vi "Digital Output.vi"(8 "error in":errorcluster, 11 "DAQmx OutPut Setting":T1) -> (0 "error out":errorcluster, 1 "Exit":bool)   [LabVIEW 2015]
uses:
  <vilib>/DAQmx/write.llb/DAQmx Write (Digital 2D Bool NChan 1Samp NLine).vi
  <vilib>/DAQmx/write.llb/DAQmx Write (Digital 1D Bool 1Chan 1Samp).vi
  <vilib>/DAQmx/create/channels.llb/DAQmx Create Channel (DO-Digital Output).vi
  Galobal variable_TI.vi
  <vilib>/DAQmx/miscellaneous.llb/DAQmx Fill In Error Info.vi
panel:
  out "array":tag[](array[tag])
  out "*(type *) &x":tag
  out "Digital Output":bool[](array[boolean])
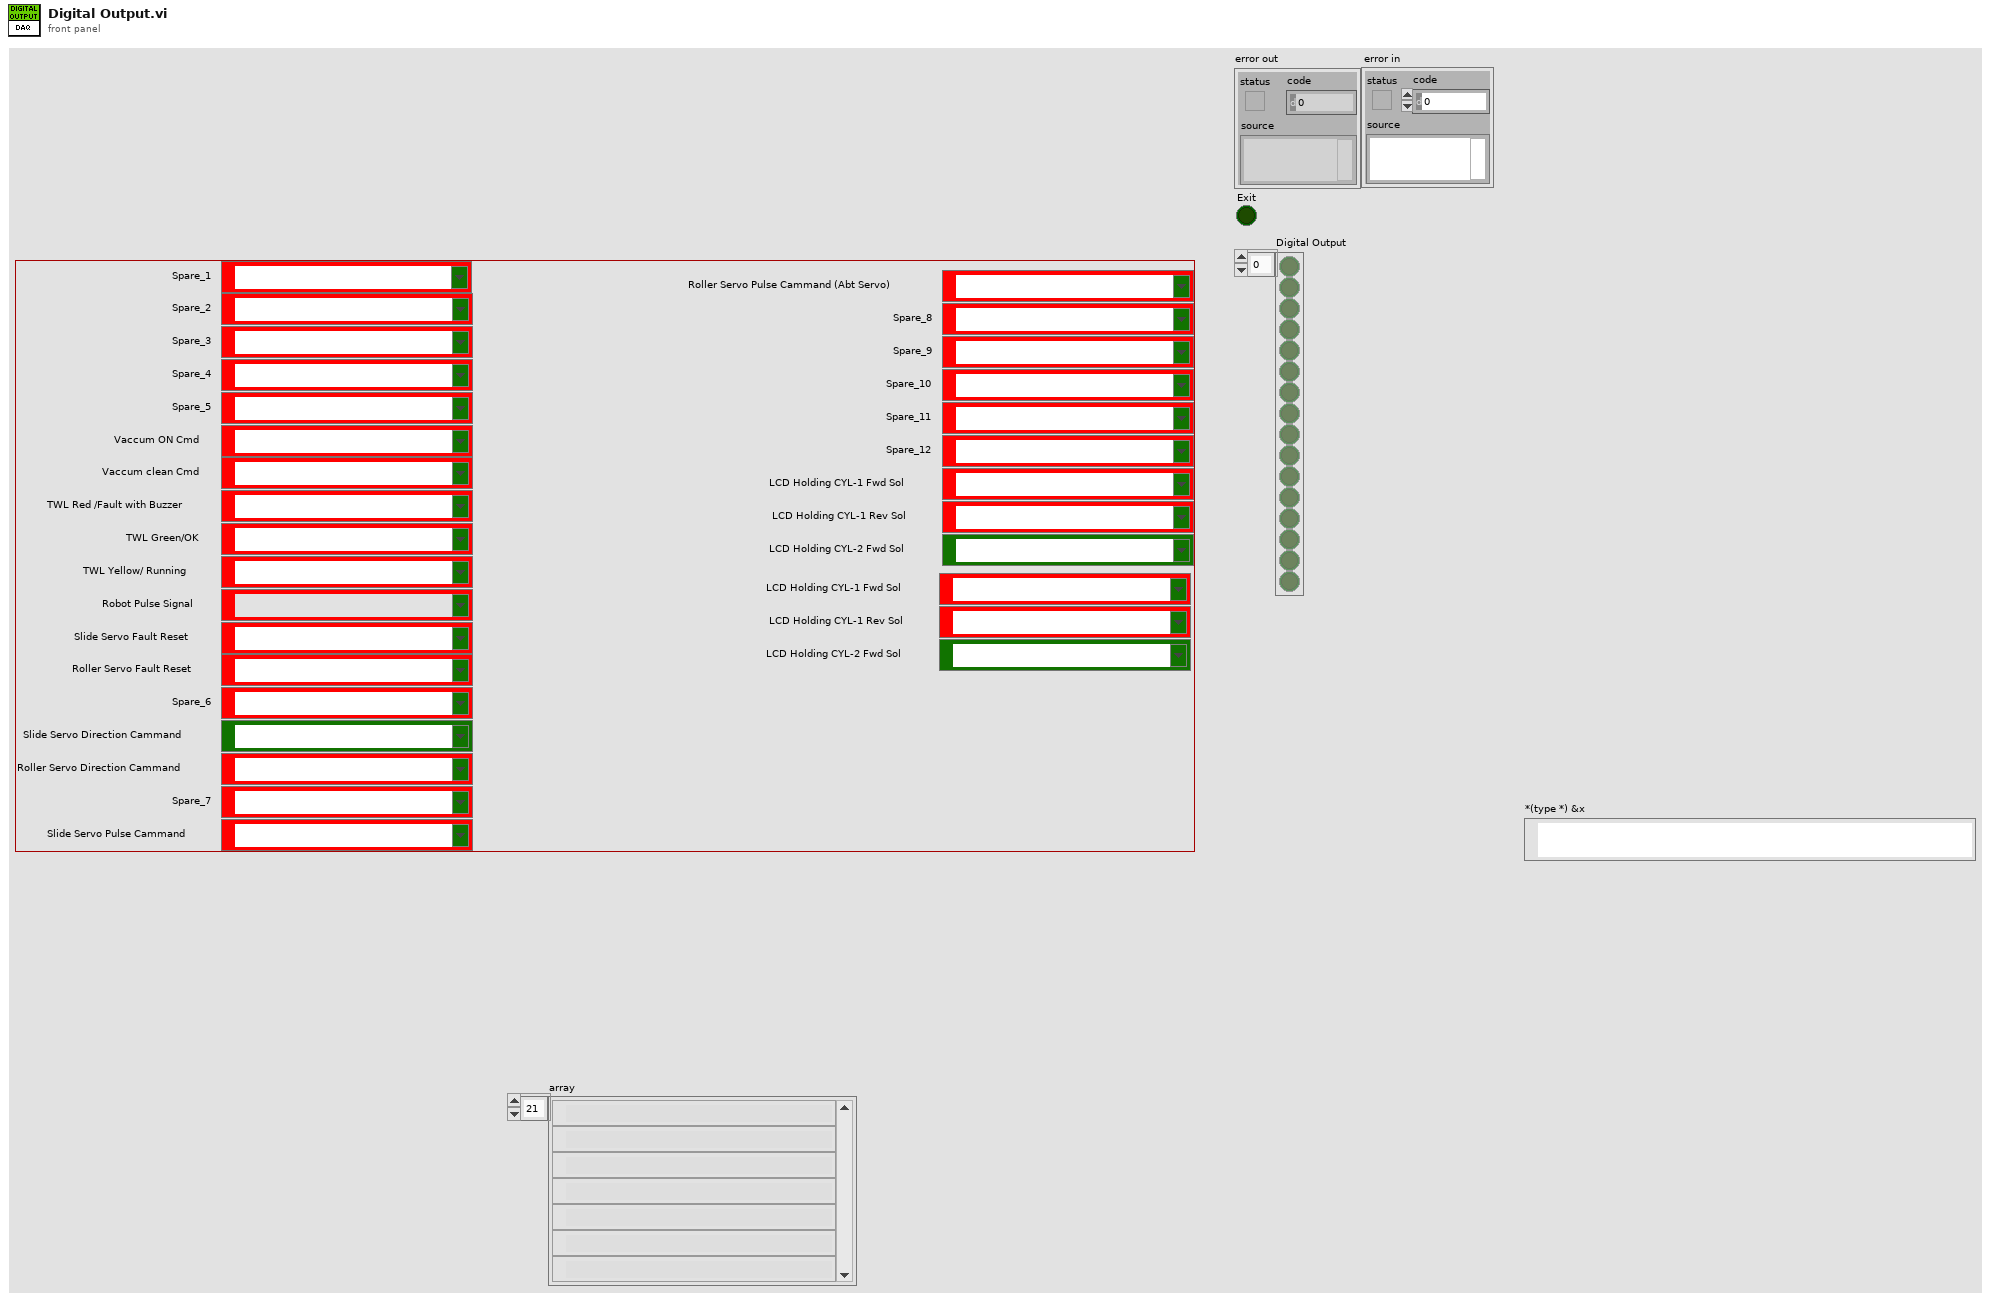
[diagram p1: front panel]
types:
  T1 = cluster{"DAQmx OutPut_00":tag, "DAQmx OutPut_01":tag, "DAQmx OutPut_02":tag, "DAQmx OutPut_03":tag, "DAQmx OutPut_04":tag, "DAQmx OutPut_05":tag, "DAQmx OutPut_06":tag, "DAQmx OutPut_07":tag, "DAQmx OutPut_08":tag, "DAQmx OutPut_09":tag, "DAQmx OutPut_10":tag, "DAQmx OutPut_11":tag, "DAQmx OutPut_12":tag, "DAQmx OutPut_13":tag, "DAQmx OutPut_14":tag, "DAQmx OutPut_15":tag, "DAQmx OutPut_16":tag, "DAQmx OutPut_17":tag, "DAQmx OutPut_18":tag, "DAQmx OutPut_19":tag, "DAQmx OutPut_20":tag, "DAQmx OutPut_21":tag, "DAQmx OutPut_22":tag, "DAQmx OutPut_23":tag, "DAQmx OutPut_12 2":tag, "DAQmx OutPut_13 2":tag, "DAQmx OutPut_14 2":tag, "DAQmx OutPut_12 3":tag, "DAQmx OutPut_13 3":tag, "DAQmx OutPut_14 3":tag}
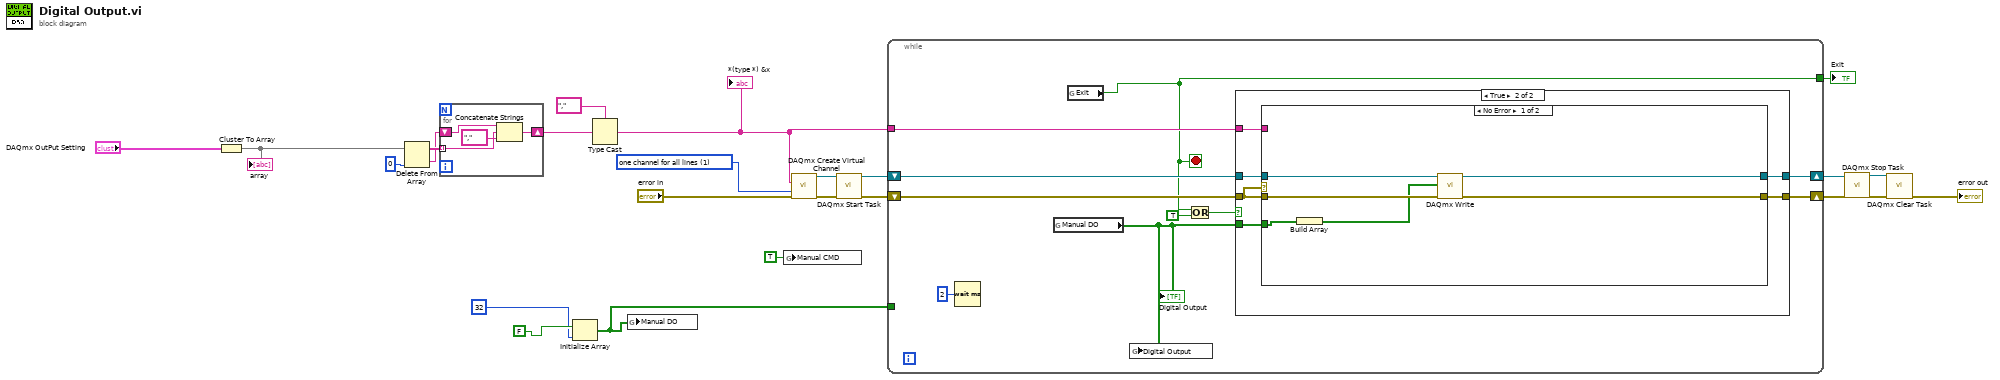
[diagram p0: block diagram]
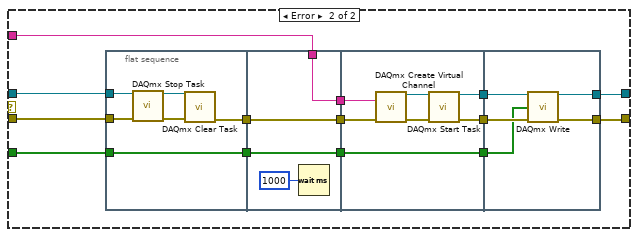
[diagram p3: hidden frame]
diagram:
  w8 = 1 items=["one channel for each line", "one channel for all lines"] ("line grouping")
  n1 = Cluster To Array(cluster="DAQmx OutPut Setting") -> (array=w6:tag[])
  "array" <- w6
  n2 = Delete From Array(array=w6, index=0) -> (deleted portion=w11:tag, array with subset deleted=w13:tag[])  [unwired: 1 in]
  n3 = for {
    tunnel: w13 -> [w27] mode=indexing
    shift-right: [w25] -> w9
    shift-left: w11 -> [w28]
    n4 = Concatenate Strings(w28, tag "," ("1."), w27) -> (w25:string)
  }
  n5 = Initialize Array(FALSE, u16 32 ("element")) -> (w1:bool[])
  n6 = Type Cast(type=tag "," ("1."), x=w9) -> (*(type *) &x=w7:tag)
  "*(type *) &x" <- w7
  n7 = global write "Galobal variable_TI.vi" "Manual DO"(w1) -> ()
  n8 = global write "Galobal variable_TI.vi" "Manual CMD"(TRUE ("Manual CMD")) -> ()
  n9 = call-poly <vilib>:"DAQmx Create Virtual Channel.vi"("lines"=w7, "line grouping"=w8, "error in"="error in") -> ("task out"=w24:refnum<k21>, "error out"=w23:errorcluster)  [unwired: 2 in, 9 out]
  n10 = call <vilib>:"DAQmx Start Task.vi"("task/channels in"=w24, "error in"=w23) -> ("task out"=w20:refnum<k21>, "error out"=w19:errorcluster)  [unwired: 12 out]
  n11 = while {
    shift-right: [w36] -> w17
    shift-left: w19 -> [w35]
    shift-right: [w37] -> w18
    shift-left: w20 -> [w38]
    tunnel: w7 -> [w34]
    tunnel: [w31] -> w14
    tunnel: w1 -> [_]
    stop <- w31 stop-if-true
    n12 = Wait (ms)(milliseconds to wait=u32 2) -> ()  [unwired: 1 out]
    n13 = global read "Galobal variable_TI.vi" "Manual DO"() -> (w30:bool[])
    "Digital Output" <- w30
    n14 = global read "Galobal variable_TI.vi" "Exit"() -> (w31:bool)
    n15 = global write "Galobal variable_TI.vi" "Digital Output"(w30) -> ()
    n16 = Or(x=w31, y=TRUE) -> (x .or. y?=w33:bool)
    n17 = case shown="True" w33 {
      tunnel: w38 -> [w40 w46]
      tunnel: [w40 w45] -> w37
      tunnel: [w39 w44] -> w36
      tunnel: w35 -> [w39 w43]
      tunnel: w34 -> [_ w42]
      tunnel: w30 -> [_ w41]
      frame False {
      }
      frame True {
        n18 = case shown="No Error" w43 {
          tunnel: w46 -> [w52 w66]
          tunnel: w43 -> [w51 w65]
          tunnel: [w50 w63] -> w45
          tunnel: [w49 w64] -> w44
          tunnel: w42 -> [_ w59]
          tunnel: w41 -> [w48 w56]
          frame No Error {
            n19 = Build Array(w48) -> (w47:bool[][])
            n20 = call-poly <vilib>:"DAQmx Write.vi"("task/channels in"=w52, "data"=w47, "error in"=w51) -> ("task out"=w50:refnum<k21>, "error out"=w49:errorcluster)  [unwired: 1 in, 10 out]
          }
          frame Error {
            n21 = flat-sequence {
              tunnel: w66 -> [w70]
              tunnel: w65 -> [w69]
              tunnel: [w68] -> w61
              tunnel: w56 -> [w67]
              tunnel: [w67] -> w55
              tunnel: [w75] -> w62
              tunnel: w61 -> [w75]
              tunnel: [w74] -> w60
              tunnel: w59 -> [w74]
              tunnel: w55 -> [w73]
              tunnel: [w73] -> w54
              tunnel: w62 -> [w79]
              tunnel: w60 -> [w78]
              tunnel: [w81] -> w58
              tunnel: [w80] -> w57
              tunnel: w54 -> [w77]
              tunnel: [w77] -> w53
              tunnel: [w86] -> w63
              tunnel: [w87] -> w64
              tunnel: w58 -> [w88]
              tunnel: w57 -> [w85]
              tunnel: w53 -> [w84]
              frame #0 {
                n22 = call <vilib>:"DAQmx Stop Task.vi"("task/channels in"=w70, "error in"=w69) -> ("task out"=w71:refnum<k21>, "error out"=w72:errorcluster)  [unwired: 12 out]
                n23 = call <vilib>:"DAQmx Clear Task.vi"("task in"=w71, "error in"=w72) -> ("error out"=w68:errorcluster)  [unwired: 13 out]
              }
              frame #1 {
                n24 = Wait (ms)(milliseconds to wait=u32 1000) -> ()  [unwired: 1 out]
              }
              frame #2 {
                n25 = call-poly <vilib>:"DAQmx Create Virtual Channel.vi"("lines"=w78, "error in"=w79) -> ("task out"=w83:refnum<k21>, "error out"=w82:errorcluster)  [unwired: 3 in, 9 out]
                n26 = call <vilib>:"DAQmx Start Task.vi"("task/channels in"=w83, "error in"=w82) -> ("task out"=w80:refnum<k21>, "error out"=w81:errorcluster)  [unwired: 12 out]
              }
              frame #3 {
                n27 = call-poly <vilib>:"DAQmx Write.vi"("task/channels in"=w85, "data"=w84, "error in"=w88) -> ("task out"=w86:refnum<k21>, "error out"=w87:errorcluster)  [unwired: 1 in, 10 out]
              }
            }
          }
        }
      }
    }
  }
  "Exit" <- w14
  n28 = call <vilib>:"DAQmx Stop Task.vi"("task/channels in"=w18, "error in"=w17) -> ("task out"=w22:refnum<k21>, "error out"=w21:errorcluster)  [unwired: 12 out]
  n29 = call <vilib>:"DAQmx Clear Task.vi"("task in"=w22, "error in"=w21) -> ("error out"=→"error out":errorcluster)  [unwired: 13 out]
